vi "AutoProgram.vi"(0 "G-Code Array":string[](array[string]), 2 "INcluster":T2, 4 "error in (no error)":errorcluster) -> (5 "Next Command":string, 6 "Stop State":bool, 7 "error out":errorcluster)   [LabVIEW 2017]
uses:
  controls/QueueControl.ctl
  controls/CommandQueue.ctl
  controls/state_board_control.ctl
  global/GLOBAL_STATE.vi
panel:
  out "size(s)":i32
  out "state_board_STM1":T1=enum."Pos"
  out "# elements in queue":i32
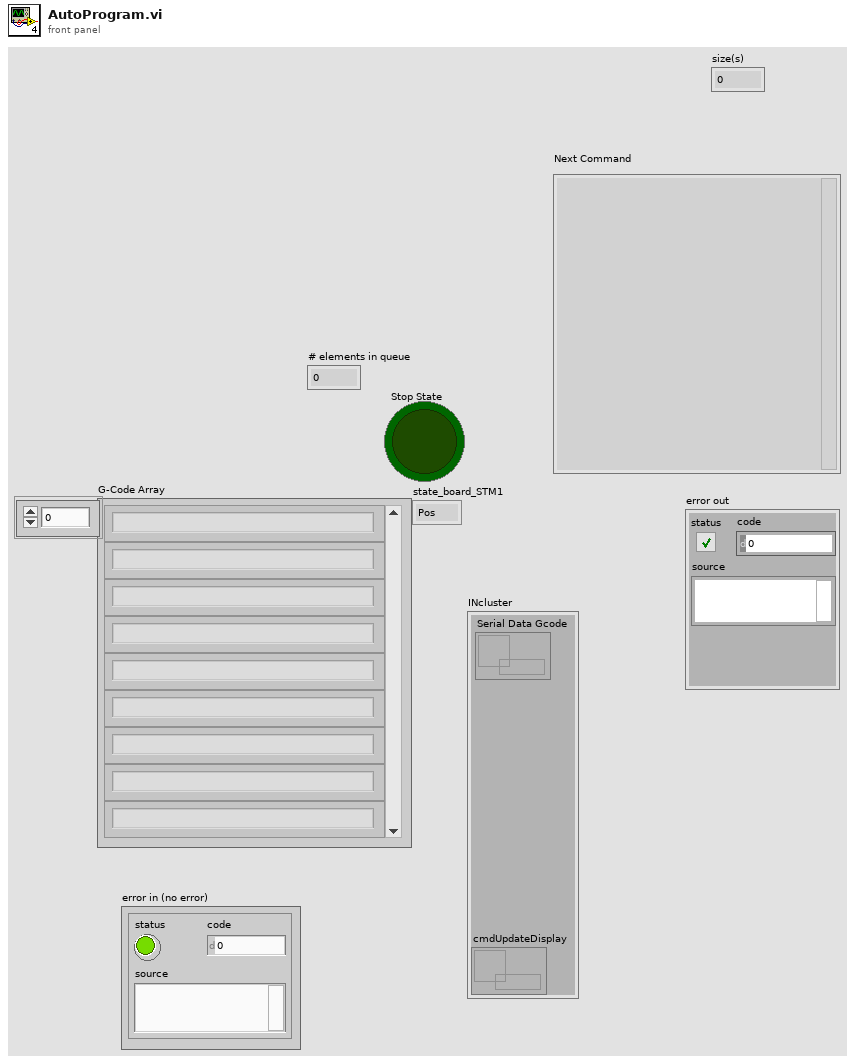
[diagram p1: front panel]
types:
  T1 = typedef "state_board_control.ctl" = enum16{"Running", "Waiting", "Pos", "IDLE"}
  T2 = typedef "QueueControl.ctl" = cluster{"Serial Data Gcode":refnum<queue>, "cmdUpdateDisplay":refnum<queue>}
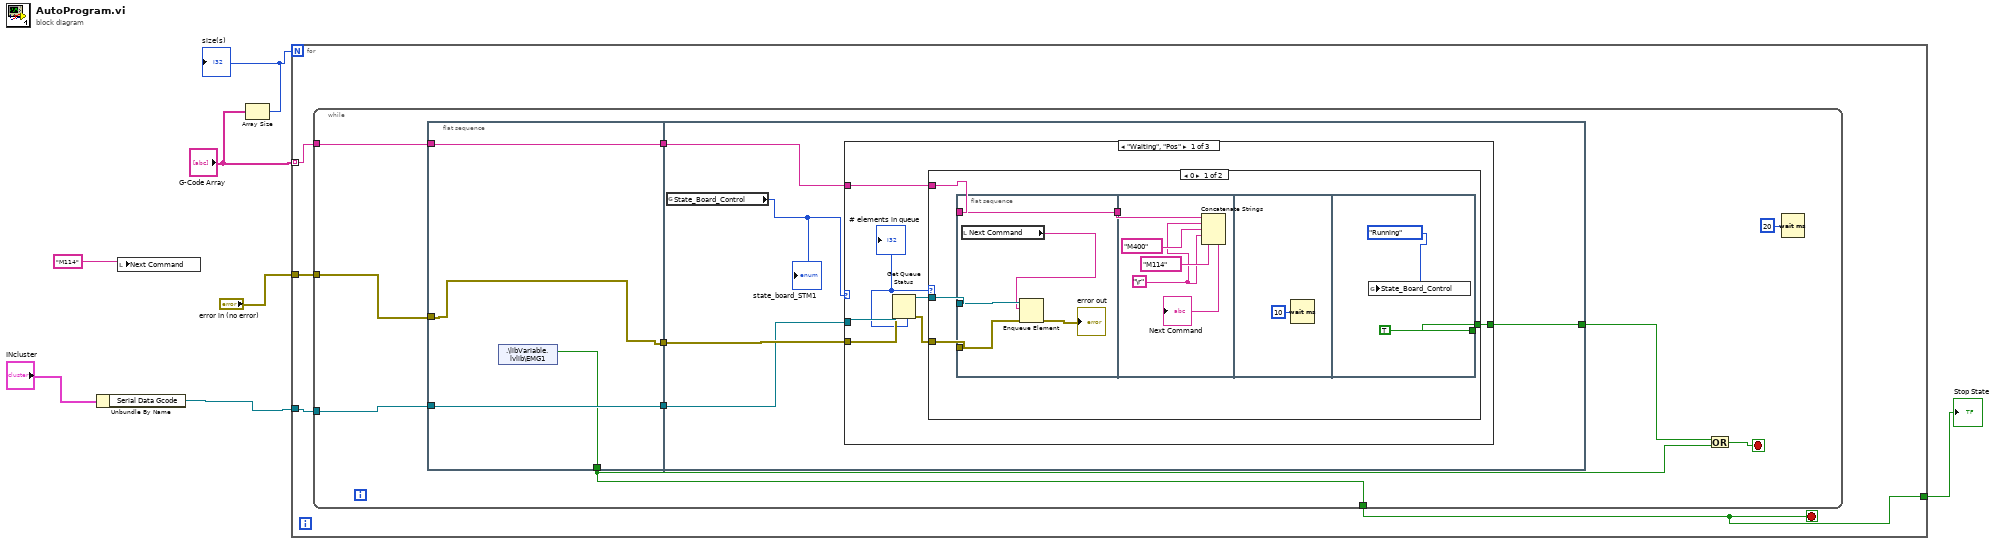
[diagram p0: block diagram]
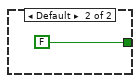
[diagram p2: hidden frame]
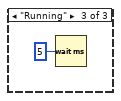
[diagram p4: hidden frame]
diagram:
  n1 = Unbundle By Name("INcluster") -> ("Serial Data Gcode"=w5:refnum<queue>)
  n2 = local write "Next Command"("M114" ("Next Command")) -> ()
  n3 = Array Size(array="G-Code Array") -> (size(s)=w1:i32)
  "size(s)" <- w1
  n4 = for {
    N: w1 -> [_]
    tunnel: "G-Code Array" -> [w9] mode=indexing
    tunnel: "error in (no error)" -> [w11]
    tunnel: w5 -> [w10]
    tunnel: [w8] -> w4
    stop <- w8 stop-if-true
    n5 = while {
      tunnel: w11 -> [w20]
      tunnel: [w18] -> w8
      tunnel: w10 -> [w16]
      tunnel: w9 -> [w15]
      stop <- w21 stop-if-true
      n6 = flat-sequence {
        tunnel: [w23] -> w19
        tunnel: [w22] -> w18
        tunnel: [w25] -> w17
        tunnel: [w24] -> w14
        tunnel: w20 -> [w23]
        tunnel: w16 -> [w25]
        tunnel: w15 -> [w24]
        tunnel: w19 -> [w30]
        tunnel: [w29] -> w12
        tunnel: w17 -> [w27]
        tunnel: w14 -> [w28]
        frame #0 {
          n7 = shared-variable ".\\libVariable.lvlib\\EMG1"() -> (w22:bool)  [unwired: 1 in, 1 out]
        }
        frame #1 {
          n8 = global read "GLOBAL_STATE.vi" "State_Board_Control"() -> (w26:T1)
          "state_board_STM1" <- w26
          n9 = case shown="\"Waiting\", \"Pos\"" w26 {
            tunnel: w27 -> [w35 _ _]
            tunnel: w30 -> [w33 _ _]
            tunnel: w28 -> [w36 _ _]
            tunnel: [w37 _ _] -> w29
            frame "Waiting", "Pos" {
              n10 = Get Queue Status(queue=w35, error in (no error)=w33) -> (queue out=w34:refnum<queue>, error out=w32:errorcluster, # elements in queue=w31:i32)  [unwired: 1 in, 5 out]
              "# elements in queue" <- w31
              n11 = case shown="0" w31 {
                tunnel: [w41 FALSE] -> w37
                tunnel: w36 -> [w38 _]
                tunnel: w34 -> [w40 _]
                tunnel: w32 -> [w39 _]
                frame 0 {
                  n12 = flat-sequence {
                    tunnel: w39 -> [w47]
                    tunnel: w38 -> [w45]
                    tunnel: [w45] -> w42
                    tunnel: w40 -> [w44]
                    tunnel: w42 -> [w51]
                    tunnel: [TRUE] -> w41
                    frame #0 {
                      n13 = local read "Next Command"() -> (w43:string)
                      n14 = Enqueue Element(queue=w44, element=w43, error in (no error)=w47) -> (error out=→"error out":errorcluster)  [unwired: 1 in, 2 out]
                    }
                    frame #1 {
                      w48 = "\r"
                      n15 = Concatenate Strings(w51, w48, "M400" ("string"), w48, "M114" ("string")) -> (→"Next Command":string)
                    }
                    frame #2 {
                      n16 = Wait (ms)(milliseconds to wait=u32 10) -> ()  [unwired: 1 out]
                    }
                    frame #3 {
                      n17 = global write "GLOBAL_STATE.vi" "State_Board_Control"(state_board_control."Running" ("state_board_STM1")) -> ()
                    }
                  }
                }
                frame Default {
                }
              }
            }
            frame "IDLE", Default {
            }
            frame "Running" {
              n18 = Wait (ms)(milliseconds to wait=u32 5) -> ()  [unwired: 1 out]
            }
          }
        }
      }
      n19 = Or(x=w12, y=w18) -> (x .or. y?=w21:bool)
      n20 = Wait (ms)(milliseconds to wait=u32 20) -> ()  [unwired: 1 out]
    }
  }
  "Stop State" <- w4
